vi "Message Type Conversion.vi"(0 "Data Type":T1, 5 "Data Length":u8, 7 "Message In":string) -> (4 "Pass/Fail?":bool, 8 "Message Out":string)   [LabVIEW 2023]
uses:
  type defs/Data Type.ctl
  library/GEA2_Toolkit.lvlib
panel:
  out "length":i32
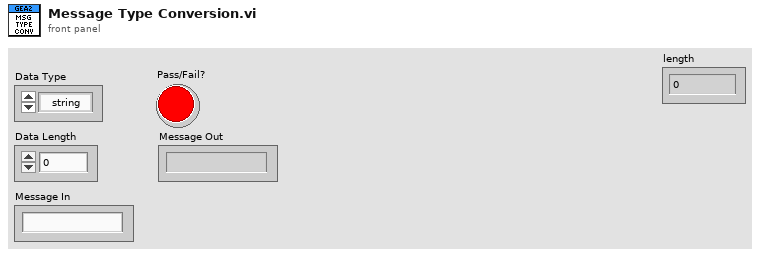
[diagram p1: front panel]
types:
  T1 = typedef "Data Type.ctl" = enum16{"string", "boolean", "uint8_t", "uint16_t", "uint32_t", "uint64_t", "int8_t", "int16_t", "int32_t", "int64_t"}
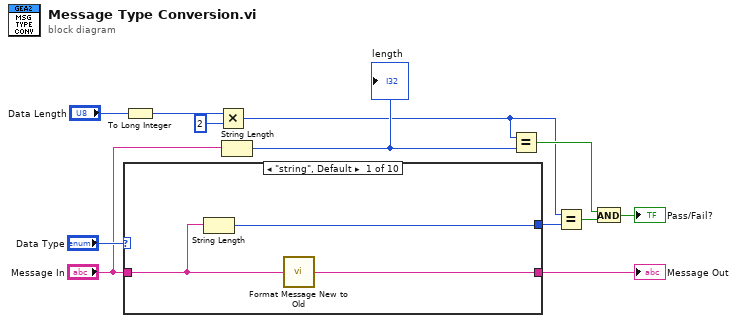
[diagram p0: block diagram]
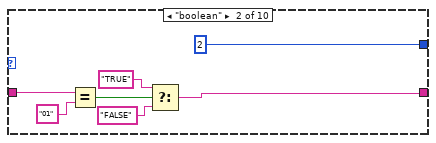
[diagram p2: hidden frame]
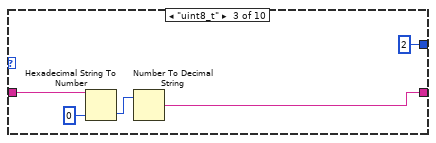
[diagram p3: hidden frame]
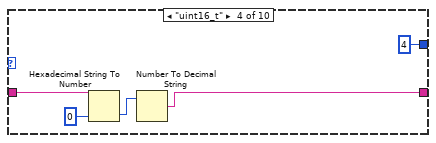
[diagram p4: hidden frame]
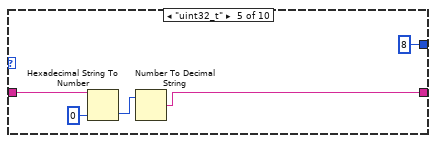
[diagram p5: hidden frame]
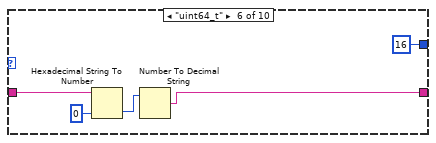
[diagram p6: hidden frame]
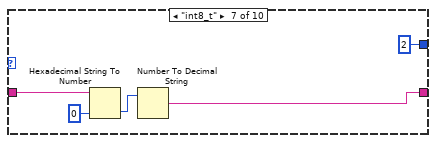
[diagram p7: hidden frame]
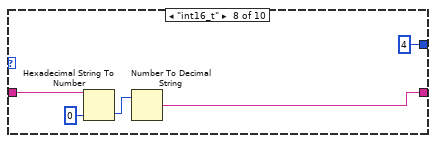
[diagram p8: hidden frame]
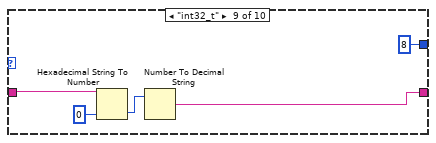
[diagram p9: hidden frame]
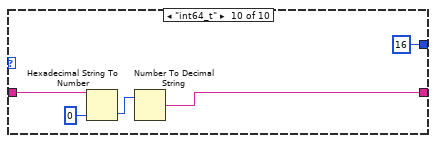
[diagram p10: hidden frame]
diagram:
  n1 = case shown="\"string\", Default" "Data Type" {
    tunnel: "Message In" -> [w14 w17 w24 w29 w34 w39 w44 w49 w53 w58]
    tunnel: [w13 w18 w26 w31 w36 w41 w46 w51 w56 w61] -> w11
    tunnel: [w15 2 ("x") 2 ("x") 4 ("x") 8 ("x") 16 ("x") 2 ("x") 4 ("x") 8 ("x") 16 ("x")] -> w9
    frame "string", Default {
      n2 = String Length(string=w14) -> (length=w15:i32)
      n3 = call "Format Message New to Old.vi"("Raw Message In"=w14) -> ("Conv Message Out"=w13:string)  [unwired: 14 in]
    }
    frame "boolean" {
      n4 = Equal?(x=w17, y="01") -> (x = y?=w21:bool)
      n5 = Select(t="TRUE", s=w21, f="FALSE") -> (s? t:f=w18:string)
    }
    frame "uint8_t" {
      n6 = Hexadecimal String To Number(string=w24, default (0uL)=u8 0) -> (number=w25:u8)  [unwired: 1 in, 1 out]
      n7 = Number To Decimal String(number=w25) -> (decimal integer string=w26:string)  [unwired: 1 in]
    }
    frame "uint16_t" {
      n8 = Hexadecimal String To Number(string=w29, default (0uL)=u16 0) -> (number=w30:u16)  [unwired: 1 in, 1 out]
      n9 = Number To Decimal String(number=w30) -> (decimal integer string=w31:string)  [unwired: 1 in]
    }
    frame "uint32_t" {
      n10 = Hexadecimal String To Number(string=w34, default (0uL)=u32 0) -> (number=w35:u32)  [unwired: 1 in, 1 out]
      n11 = Number To Decimal String(number=w35) -> (decimal integer string=w36:string)  [unwired: 1 in]
    }
    frame "uint64_t" {
      n12 = Hexadecimal String To Number(string=w39, default (0uL)=u64 0) -> (number=w40:u64)  [unwired: 1 in, 1 out]
      n13 = Number To Decimal String(number=w40) -> (decimal integer string=w41:string)  [unwired: 1 in]
    }
    frame "int8_t" {
      n14 = Hexadecimal String To Number(string=w44, default (0uL)=i8 0) -> (number=w45:i8)  [unwired: 1 in, 1 out]
      n15 = Number To Decimal String(number=w45) -> (decimal integer string=w46:string)  [unwired: 1 in]
    }
    frame "int16_t" {
      n16 = Hexadecimal String To Number(string=w49, default (0uL)=i16 0) -> (number=w50:i16)  [unwired: 1 in, 1 out]
      n17 = Number To Decimal String(number=w50) -> (decimal integer string=w51:string)  [unwired: 1 in]
    }
    frame "int32_t" {
      n18 = Hexadecimal String To Number(string=w53, default (0uL)=0) -> (number=w55:i32)  [unwired: 1 in, 1 out]
      n19 = Number To Decimal String(number=w55) -> (decimal integer string=w56:string)  [unwired: 1 in]
    }
    frame "int64_t" {
      n20 = Hexadecimal String To Number(string=w58, default (0uL)=i64 0) -> (number=w60:i64)  [unwired: 1 in, 1 out]
      n21 = Number To Decimal String(number=w60) -> (decimal integer string=w61:string)  [unwired: 1 in]
    }
  }
  "Message Out" <- w11
  n22 = To Long Integer(number="Data Length") -> (32bit integer=w1:i32)
  n23 = Multiply(x=w1, y=2) -> (x*y=w3:i32)
  n24 = String Length(string="Message In") -> (length=w8:i32)
  "length" <- w8
  n25 = Equal?(x=w3, y=w8) -> (x = y?=w6:bool)
  n26 = Equal?(x=w3, y=w9) -> (x = y?=w7:bool)
  n27 = And(x=w6, y=w7) -> (x .and. y?=→"Pass/Fail?":bool)
